vi "Analysis.Result Summaries, Generate Yield Per Day_V2.vi"(9 "Type":enum16{"First Pass", "Last Pass", "All"}(ring), 11 "ResultSum":T1[](array[typedef])) -> (2 "Yield Per Date":string[][](table), 3 "Yield vs Date":cluster{timestamp[], dbl[]}(graph))   [LabVIEW 2024]
uses:
  Analysis.Result Summary.ctl
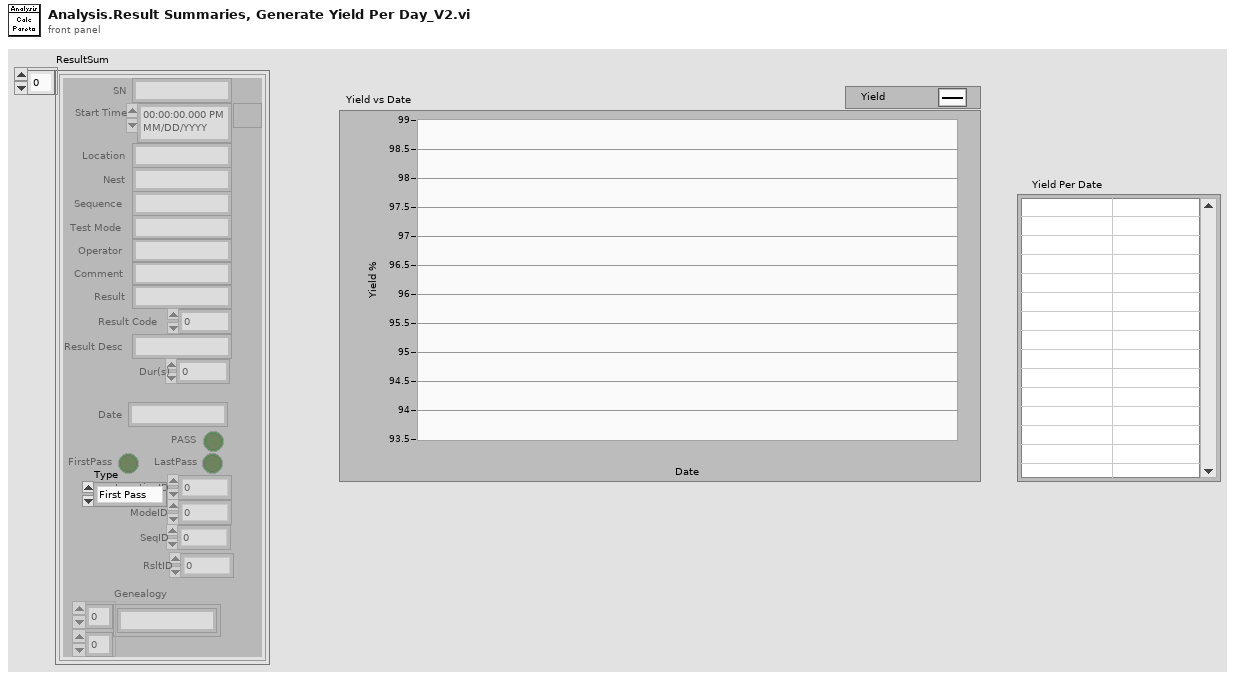
[diagram p1: front panel]
types:
  T1 = typedef "Analysis.Result Summary.ctl" = cluster{"SN":string, "Start Time":timestamp, "Location":string, "Nest":string, "Sequence":string, "Operator":string, "Test Mode":string, "Comment":string, "Result":string, "Result Code":i32, "Result Desc":string, "Date":string, "Dur(s)":dbl, "PASS":bool, "FirstPass":bool, "LastPass":bool, "LocationID":i32, "ModeID":i32, "SeqID":i32, "RsltID":i32, "Genealogy":string[][]}
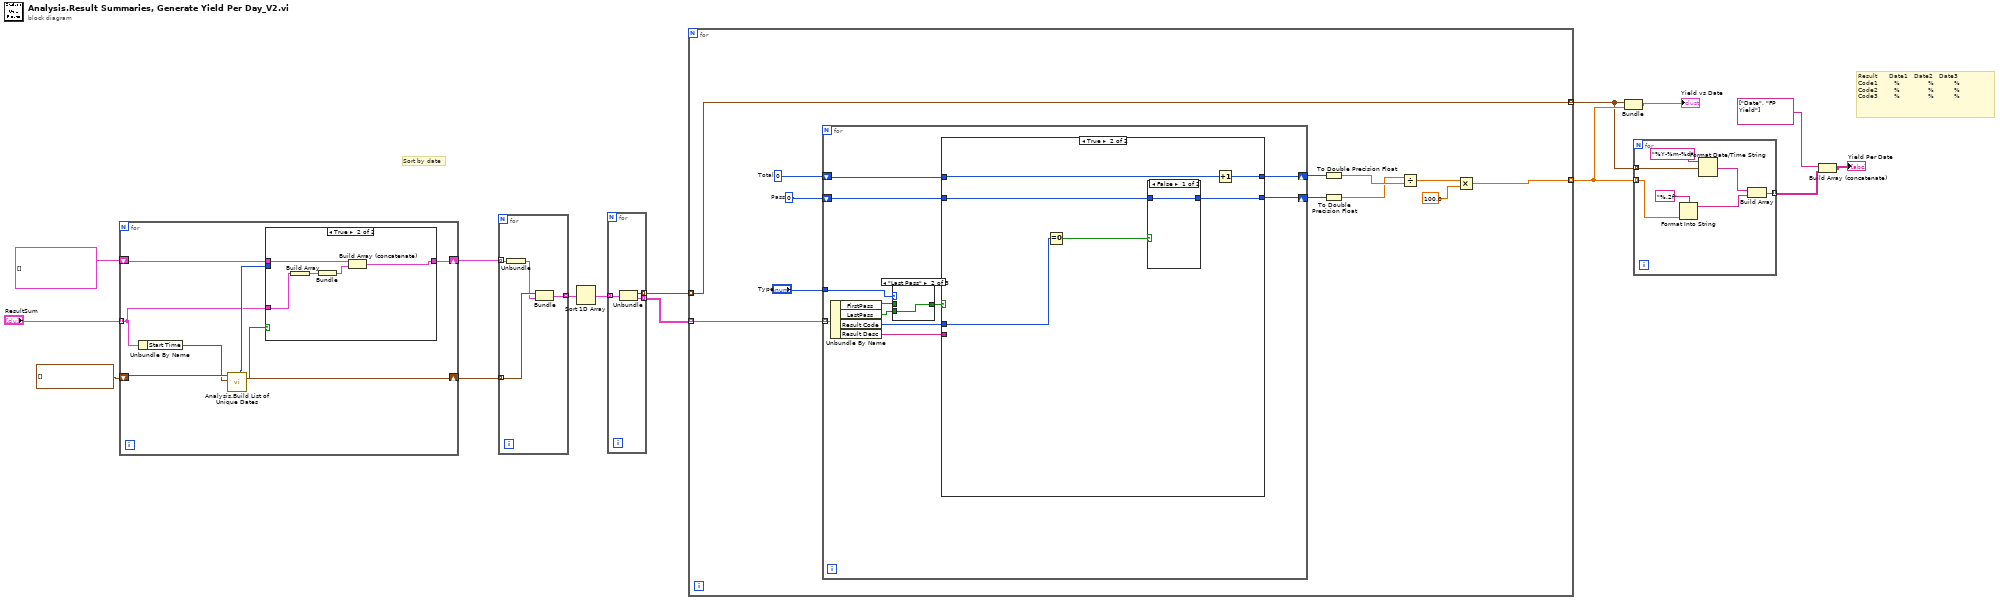
[diagram p0: block diagram]
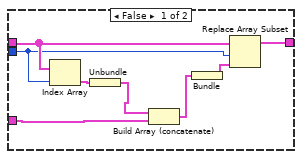
[diagram p2: hidden frame]
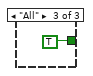
[diagram p4: hidden frame]
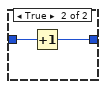
[diagram p6: hidden frame]
diagram:
  # "Sort by date"
  # "Result      Date1   Date2   Date3                 \nCode1        %              %          %\nCode2        %              %          %\nCode3        %              %          %"
  n1 = for {
    tunnel: "ResultSum" -> [w20] mode=indexing
    shift-right: [w22] -> w12
    shift-left: timestamp[] [] -> [w23]
    shift-right: [w17] -> w13
    shift-left: cluster{"ResultSum":T1[]}[] [] ("ResultSum") -> [w19]
    n2 = Unbundle By Name(w20) -> ("Start Time"=w16:timestamp)
    n3 = call "Analysis.Build List of Unique Dates.vi"("Date In"=w16, "Dates In"=w23) -> ("Added"=w18:bool, "Dates Out"=w22:timestamp[], "Index"=w21:i32)  [unwired: 7 in]
    n4 = case shown="True" w18 {
      tunnel: w21 -> [w30 _]
      tunnel: w20 -> [w29 w34]
      tunnel: w19 -> [w31 w36]
      tunnel: [w24 w35] -> w17
      frame False {
        n5 = Index Array(array=w31, index=w30) -> (element=w28:cluster{"ResultSum":T1[]})
        n6 = Unbundle(w28) -> ("ResultSum"=w27:T1[])
        n7 = Build Array (concatenate)(w27, w29) -> (w26:T1[])
        n8 = Bundle(w26) -> (w25:cluster{T1[]})  [unwired: 1 in]
        n9 = Replace Array Subset(array=w31, new element=w25, index=w30) -> (w24:cluster{"ResultSum":T1[]}[])
      }
      frame True {
        n10 = Build Array(w34) -> (w33:T1[])
        n11 = Bundle(w33) -> (w32:cluster{T1[]})  [unwired: 1 in]
        n12 = Build Array (concatenate)(w36, w32) -> (w35:cluster{"ResultSum":T1[]}[])
      }
    }
  }
  n13 = for {
    tunnel: w13 -> [w38] mode=indexing
    tunnel: w12 -> [w40] mode=indexing
    tunnel: [w39] -> w11 mode=indexing
    n14 = Unbundle(w38) -> ("ResultSum"=w37:T1[])
    n15 = Bundle("String"=w40, "ResultSum"=w37) -> (w39:cluster{"String":timestamp, "ResultSum":T1[]})  [unwired: 1 in]
  }
  n16 = Sort 1D Array(array=w11) -> (sorted array=w10:cluster{"String":timestamp, "ResultSum":T1[]}[])
  n17 = for {
    tunnel: w10 -> [w43] mode=indexing
    tunnel: [w42] -> w9 mode=indexing
    tunnel: [w41] -> w7 mode=indexing
    n18 = Unbundle(w43) -> ("String"=w41:timestamp, "ResultSum"=w42:T1[])
  }
  n19 = for {
    tunnel: w9 -> [w54] mode=indexing
    tunnel: w7 -> [w52] mode=indexing
    tunnel: [w52] -> w4 mode=indexing
    tunnel: [w44] -> w5 mode=indexing
    w51 = 0  # Pass
    w55 = 0  # Total
    n20 = for {
      shift-right: [w65] -> w49
      shift-left: w51 -> [w66]
      tunnel: w54 -> [w62] mode=indexing
      shift-right: [w63] -> w50
      shift-left: w55 -> [w64]
      tunnel: "Type" -> [w60]
      n21 = Unbundle By Name(w62) -> ("FirstPass"=w59:bool, "LastPass"=w58:bool, "Result Code"=w56:i32, "Result Desc"=w61:string)
      n22 = case shown="\"Last Pass\"" w60 {
        tunnel: w59 -> [w67 _ _]
        tunnel: w58 -> [_ w68 _]
        tunnel: [w67 w68 TRUE] -> w57
        frame "First Pass", Default {
        }
        frame "Last Pass" {
        }
        frame "All" {
        }
      }
      n23 = case shown="True" w57 {
        tunnel: w66 -> [w70 w73]
        tunnel: [w70 w72] -> w65
        tunnel: w64 -> [w71 w76]
        tunnel: [w71 w77] -> w63
        tunnel: w56 -> [_ w75]
        tunnel: w61 -> [_ _]
        frame False {
        }
        frame True {
          n24 = Equal To 0?(x=w75) -> (x = 0?=w74:bool)
          n25 = case shown="False" w74 {
            tunnel: w73 -> [w78 w80]
            tunnel: [w78 w79] -> w72
            frame False {
            }
            frame True {
              n26 = Increment(x=w80) -> (x+1=w79:i32)
            }
          }
          n27 = Increment(x=w76) -> (x+1=w77:i32)
        }
      }
    }
    n28 = To Double Precision Float(number=w50) -> (double precision float=w48:dbl)
    n29 = To Double Precision Float(number=w49) -> (double precision float=w47:dbl)
    n30 = Divide(x=w47, y=w48) -> (x/y=w46:dbl)
    n31 = Multiply(x=w46, y=100.0) -> (x*y=w44:dbl)
  }
  n32 = Bundle(w4, w5) -> (→"Yield vs Date":cluster{timestamp[], dbl[]})  [unwired: 1 in]
  n33 = for {
    tunnel: w5 -> [w85] mode=indexing
    tunnel: w4 -> [w87] mode=indexing
    tunnel: [w81] -> w3 mode=indexing
    n34 = Format Into String(format string="%.2f", w85) -> (resulting string=w82:string)  [unwired: 2 in, 1 out]
    n35 = Format Date/Time String(time format string (%c)="%Y-%m-%d", seconds (now)=w87) -> (date/time string=w83:string)  [unwired: 1 in]
    n36 = Build Array(w83, w82) -> (w81:string[])
  }
  n37 = Build Array (concatenate)(string[] ["Date", "FP Yield"], w3) -> (→"Yield Per Date":string[][])
